vi "PFI-28000-Chan-28144-V_Get Bridge Configuration.vi"(8 "error in (no error)":errorcluster, 11 "PFI-28000-Chan-28144-V in":refnum<class "PFI-28000-Chan-28144-V.lvclass">) -> (0 "error out":errorcluster, 2 "Bridge Configuration":T1, 3 "PFI-28000-Chan-28144-V out":refnum<class "PFI-28000-Chan-28144-V.lvclass">)   [LabVIEW 2017, in "PFI-28000-Chan-28144-V.lvclass"]
uses:
  PFI-28000-Chan-28144-V.lvclass
  C:/wc/07143 Precision Filters 28000 Support/Driver/source/Channel/PFI-28000-Channel.lvclass
  PFI-28000-Chan-28144-V-Bridge Configuration.ctl
  Utilities/PFI-28000-Utils.lvlib
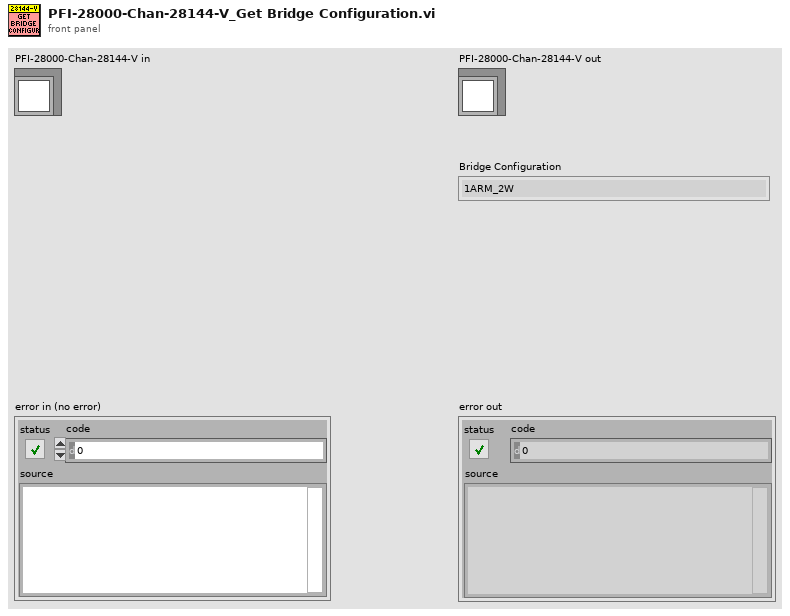
[diagram p1: front panel]
types:
  T1 = typedef "PFI-28000-Chan-28144-V.lvclass/PFI-28000-Chan-28144-V-Bridge Configuration.ctl" = enum8{"1ARM_2W", "1ARM_3W", "2ARM", "4ARM"}
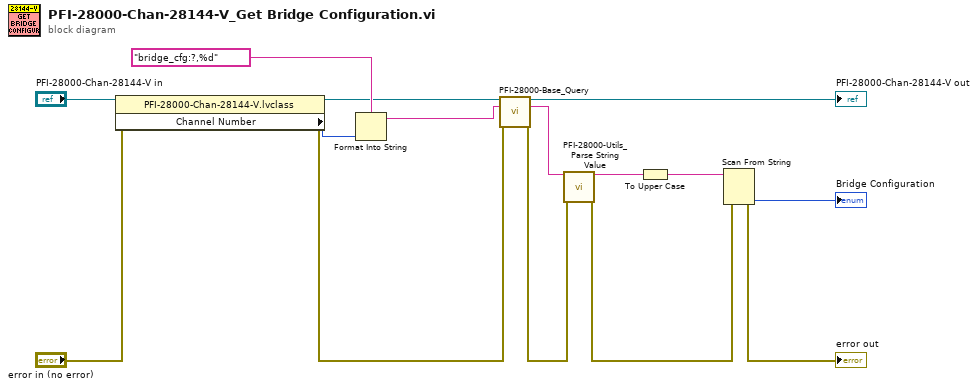
[diagram p0: block diagram]
diagram:
  n1 = property class="PFI-28000-Chan-28144-V.lvclass"(reference="PFI-28000-Chan-28144-V in", error in="error in (no error)") -> (reference out=w9:refnum<class "PFI-28000-Chan-28144-V.lvclass">, error out=w7:errorcluster, "Channel Number"=w13:i32)
  n2 = Format Into String(format string="bridge_cfg:?,%d" ("empty string"), w13) -> (resulting string=w8:string)  [unwired: 2 in, 1 out]
  n3 = call-dynamic "PFI-28000-Base_Query.vi"("PFI-28000-Base in"=w9, "Command"=w8, "error in (no error)"=w7) -> ("PFI-28000-Base out"=→"PFI-28000-Chan-28144-V out":refnum<class "PFI-28000-Chan-28144-V.lvclass">, "Response"=w4:string, "error out"=w3:errorcluster)  [unwired: 9 in, 1 out]
  n4 = call "PFI-28000-Utils_Parse String Value.vi"("String"=w4, "error in (no error)"=w3) -> ("String Value"=w5:string, "error out"=w2:errorcluster)  [unwired: 11 in, 1 out]
  n5 = To Upper Case(1:w5) -> (0:w1:string)
  n6 = Scan From String(input string=w1, error in=w2) -> (error out=→"error out":errorcluster, output 1=→"Bridge Configuration":T1)  [unwired: 3 in, 2 out]
